vi "RPi WebDAV.vi"(8 "Error IN":errorcluster, 9 "RPi Sub-Dir":string="Data/Sync", 10 "RPi IP":string="10.31.176.36", 11 "RIO Folder":path=path "u:/Data/AKLH/Sync") -> (0 "Error OUT":errorcluster={"status"=TRUE, "code"=-1967362020, "source"="NI_WebDAV.lvlib:Close Session.vi:4230001<APPEND>\n\n<b>Complete call chain:</b>\n     NI_WebDAV.lvlib:Close Session.vi:4230001\n     RPi WebDAV.vi\n     Push Sync Files to WebDAV.vi\n     Data Logger Main.vi\n     Data Logger Loop.vi\n     TI sbRIO Main (RT).vi"}, 3 "Files Paths":path[](array[path]))   [LabVIEW 2018]
uses:
  <vilib>/WebDAVClient/Advanced/Put File.vi
  <vilib>/WebDAVClient/NI_WebDAV.lvlib
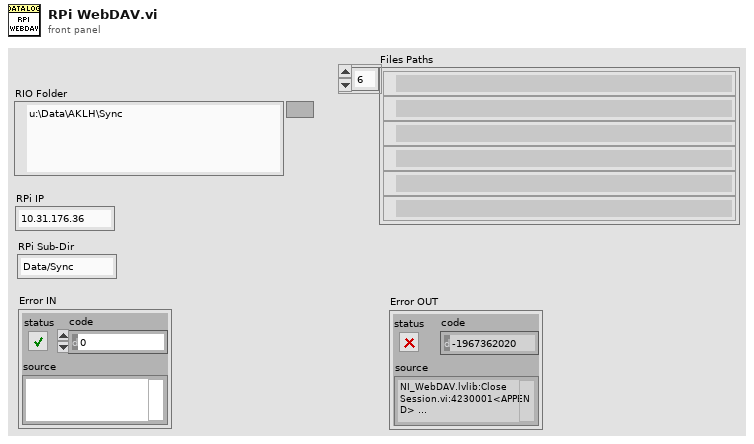
[diagram p1: front panel]
types:
  T1 = typedef "NI_WebDAV.lvlib/SessionHandle.ctl" = refnum<k1>
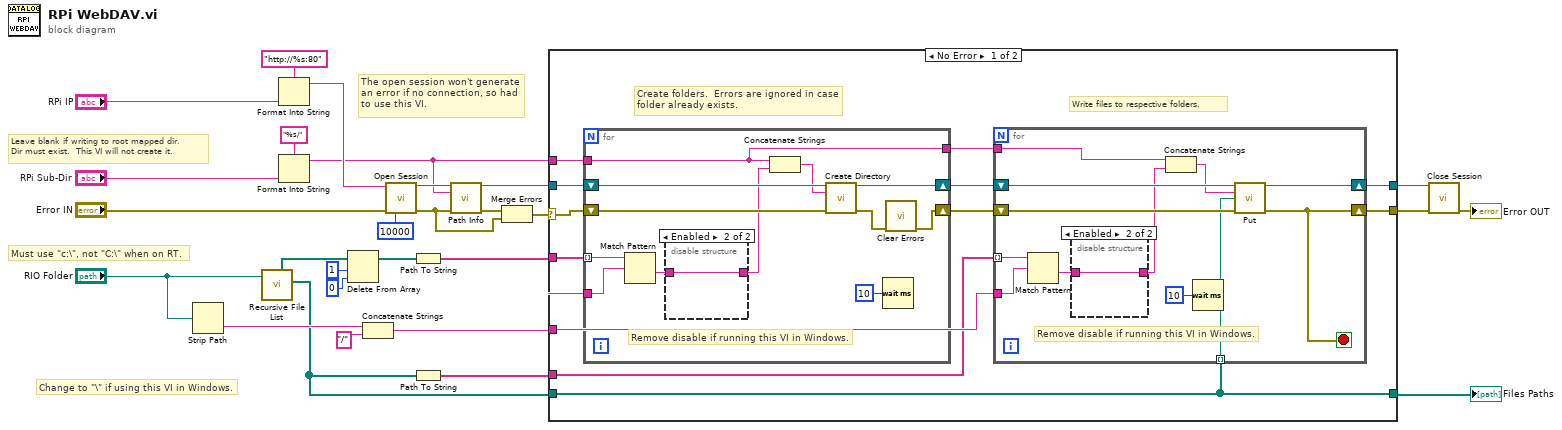
[diagram p0: block diagram]
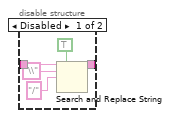
[diagram p2: hidden frame]
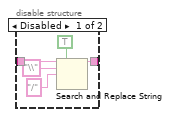
[diagram p3: hidden frame]
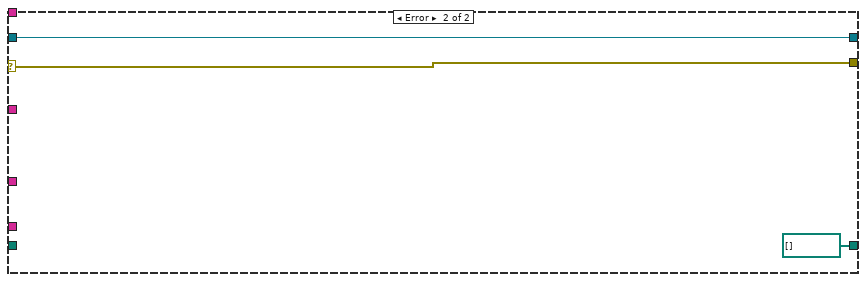
[diagram p4: hidden frame]
diagram:
  # "The open session won't generate\nan error if no connection, so had\nto use this VI."
  # "Leave blank if writing to root mapped dir.\nDir must exist.  This VI will not create it."
  # "Change to \"\\\" if using this VI in Windows."
  # "Must use \"c:\\\", not \"C:\\\" when on RT."
  n1 = Strip Path(path="RIO Folder") -> (name=w23:string)  [unwired: 1 out]
  n2 = call <vilib>:"Recursive File List.vi"("Folder Path"="RIO Folder") -> ("All Files in Dir"=w21:path[], "All Folders"=w28:path[])  [unwired: 6 in, 3 out]
  n3 = Format Into String(format string="http://%s:80" ("file uri"), "RPi IP") -> (resulting string=w16:string)  [unwired: 2 in, 1 out]
  n4 = Format Into String(format string="%s/" ("file uri"), "RPi Sub-Dir") -> (resulting string=w2:string)  [unwired: 2 in, 1 out]
  n5 = Delete From Array(array=w28, length=1, index=0) -> (array with subset deleted=w25:path[])  [unwired: 1 out]
  n6 = Concatenate Strings(w23, "/" ("format string")) -> (w22:string)
  n7 = call <vilib>:"Open Session.vi"("host uri prefix"=w16, "error in (no error)"="Error IN", "timeout ms"=10000) -> ("session handle out"=w6:T1, "error out"=w5:errorcluster)  [unwired: 11 in]
  n8 = Path To String(path=w25) -> (string=w15:string[])
  n9 = Path To String(path=w21) -> (string=w14:string[])
  n10 = call <vilib>:"Path Info.vi"("session handle"=w6, "relative uri"=w2, "error in (no error)"=w5) -> ("session handle out"=w1:T1, "error out"=w4:errorcluster)  [unwired: 9 in, 2 out]
  n11 = Merge Errors(w4, w5) -> (w3:errorcluster)
  n12 = case shown="No Error" w3 {
    selector: w3 -> [w29 w77]
    tunnel: w22 -> [w40 _]
    tunnel: w21 -> [w30 _]
    tunnel: w1 -> [w39 w79]
    tunnel: w15 -> [w38 _]
    tunnel: w14 -> [w35 _]
    tunnel: [w34 w79] -> w13
    tunnel: [w33 w77] -> w12
    tunnel: w2 -> [w32 _]
    tunnel: [w30 path[] [] ("All Files in Dir")] -> w7
    frame No Error {
      # "Write files to respective folders."
      # "Create folders.  Errors are ignored in case\nfolder already exists."
      n13 = for {
        tunnel: w38 -> [w65] mode=indexing
        tunnel: w40 -> [w64]
        tunnel: w32 -> [w60]
        tunnel: [w60] -> w31
        shift-right: [w67] -> w37
        shift-left: w39 -> [w68]
        shift-right: [w66] -> w36
        shift-left: w29 -> [w69]
        # "Remove disable if running this VI in Windows."
        n14 = Match Pattern(string=w65, regular expression=w64) -> (after substring=w63:string)  [unwired: 1 in, 3 out]
        n15 = disable-structure shown="Enabled" {
          disable-tunnel: [w75 w76] -> w62
          disable-tunnel: w63 -> [w73 w76]
          frame Disabled {
            n16 = Search and Replace String(replace all?=TRUE ("replace all? (F)"), input string=w73, search string="\\", replace string="/" ("replace string (\"\")")) -> (result string=w75:string)  [unwired: 4 in, 3 out]
          }
          frame Enabled {
          }
        }
        n17 = Concatenate Strings(w60, w62) -> (w61:string)
        n18 = call <vilib>:"Create Directory.vi"("session handle"=w68, "relative uri"=w61, "error in (no error)"=w69) -> ("session handle out"=w67:T1, "error out"=w70:errorcluster)  [unwired: 11 in]
        n19 = Wait (ms)(milliseconds to wait=u32 10) -> ()  [unwired: 1 out]
        n20 = call <vilib>:"Clear Errors.vi"("error in (no error)"=w70) -> ("error out"=w66:errorcluster)  [unwired: 5 in, 1 out]
      }
      n21 = for {
        tunnel: w35 -> [w49] mode=indexing
        tunnel: w40 -> [w48]
        tunnel: w30 -> [w47] mode=indexing
        tunnel: w31 -> [w45]
        shift-right: [w50] -> w34
        shift-left: w37 -> [w51]
        shift-right: [w42] -> w33
        shift-left: w36 -> [w52]
        stop <- w42 stop-if-true
        # "Remove disable if running this VI in Windows."
        n22 = Match Pattern(string=w49, regular expression=w48) -> (after substring=w46:string)  [unwired: 1 in, 3 out]
        n23 = disable-structure shown="Enabled" {
          disable-tunnel: [w57 w58] -> w44
          disable-tunnel: w46 -> [w55 w58]
          frame Disabled {
            n24 = Search and Replace String(replace all?=TRUE ("replace all? (F)"), input string=w55, search string="\\", replace string="/" ("replace string (\"\")")) -> (result string=w57:string)  [unwired: 4 in, 3 out]
          }
          frame Enabled {
          }
        }
        n25 = Concatenate Strings(w45, w44) -> (w43:string)
        n26 = Wait (ms)(milliseconds to wait=u32 10) -> ()  [unwired: 1 out]
        n27 = call-poly <vilib>:"Put.vi"("session handle"=w51, "relative uri"=w43, "local file path"=w47, "error in (no error)"=w52) -> ("session handle out"=w50:T1, "error out"=w42:errorcluster)  [unwired: 9 in, 1 out]
      }
    }
    frame Error {
    }
  }
  "Files Paths" <- w7
  n28 = call <vilib>:"Close Session.vi"("session handle"=w13, "error in (no error)"=w12) -> ("error out"=→"Error OUT":errorcluster)  [unwired: 13 in]
